vi "Add Properties.vi"(8 "error in":errorcluster, 10 "Item in":refnum<class "Item.lvclass">, 11 "Node Ptr in":T1 format="%.0x") -> (0 "error out":errorcluster, 3 "Node Ptr out":T1 format="%.0x")   [LabVIEW 2024, in "FPGA Addon System Explorer.lvlib"]
uses:
  FPGA Addon System Explorer.lvlib
  <vilib>/NI VeriStand/Custom Device API/Custom Device Item Ref.ctl
  Parser/Item/Item.lvclass
  <vilib>/NI VeriStand/Custom Device API/Dependent File Optional Info.ctl
  Parser/Property/Get Property Data/Get Property Data (Double).vi
  <vilib>/NI VeriStand/Custom Device API/Set Item Property (Double).vi
  Parser/Property/Get Property Data/Get Property Data (Boolean).vi
  <vilib>/NI VeriStand/Custom Device API/Set Item Property (Boolean).vi
  Parser/Property/Get Property Data/Get Property Data (DoubleArray).vi
  <vilib>/NI VeriStand/Custom Device API/Set Item Property (Double Array).vi
  Parser/Property/Get Property Data/Get Property Data (StringArray).vi
  <vilib>/NI VeriStand/Custom Device API/Set Item Property (String Array).vi
  Parser/Property/Get Property Data/Get Property Data (I32).vi
  <vilib>/NI VeriStand/Custom Device API/Set Item Property (I32).vi
  Parser/Property/Get Property Data/Get Property Data (U32).vi
  <vilib>/NI VeriStand/Custom Device API/Set Item Property (U32).vi
  Parser/Property/Get Property Data/Get Property Data (U16).vi
  <vilib>/NI VeriStand/Custom Device API/Set Item Property (U16).vi
  Parser/Property/Get Property Data/Get Property Data (U64).vi
  <vilib>/NI VeriStand/Custom Device API/Set Item Property (U64).vi
  Parser/Property/Get Property Data/Get Property Data (I32Array).vi
  <vilib>/NI VeriStand/Custom Device API/Set Item Property (I32 Array).vi
  Parser/Property/Get Property Data/Get Property Data (U32Array).vi
  <vilib>/NI VeriStand/Custom Device API/Set Item Property (U32 Array).vi
  Parser/Property/Get Property Data/Get Property Data (Variant).vi
  <vilib>/NI VeriStand/Custom Device API/Set Item Property (Variant).vi
  Parser/Property/Get Property Data/Get Property Data (String).vi
  <vilib>/NI VeriStand/Custom Device API/Set Item Property (String).vi
  Parser/Property/Get Property Data/Get Property Data (Path).vi
  <vilib>/NI VeriStand/Custom Device API/Set Item Property (Path).vi
  Parser/Property/Get Property Data/Get Property Data (Dictionary).vi
  Parser/Property/Get Property Data/Get Property Data (DependentFile).vi
  <vilib>/NI VeriStand/Custom Device API/Set Item Property (Dependent File).vi
  <vilib>/NI VeriStand/Custom Device API/Custom Device API.lvlib
  Parser/Property/Property.lvclass
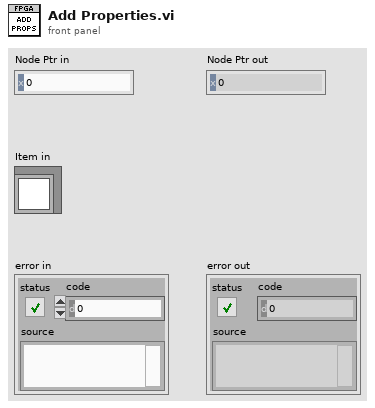
[diagram p1: front panel]
types:
  T1 = typedef "Custom Device API.lvlib/Custom Device Item Ref.ctl" = u64
  T2 = typedef "Custom Device API.lvlib/Dependent File Optional Info.ctl" = cluster{"Version":string, "RTDestination":path, "ForceDownload":bool, "SupportedTarget":string, "MD5":string}
  T3 = typedef "Parser.lvlib/Property.lvclass/Property Type.ctl" = enum16{"Boolean", "Double", "String", "Path", "Dictionary", "DependentFile", "I16", "I32", "I64", "U16", "U32", "U64", "BooleanArray", "DoubleArray", "StringArray", "I16Array", "I32Array", "I64Array", "U16Array", "U32Array", "U64Array", "Variant"}
  T4 = cluster{"Name":string, "Type":T3, "Value":variant}[]
  T5 = typedef "Parser.lvlib/Property.lvclass/DependentFile.ctl" = cluster{"Path":path, "Version":string, "RTDestination":path, "ForceDownload":bool, "SupportedTarget":string, "MD5":string, " Type":string}
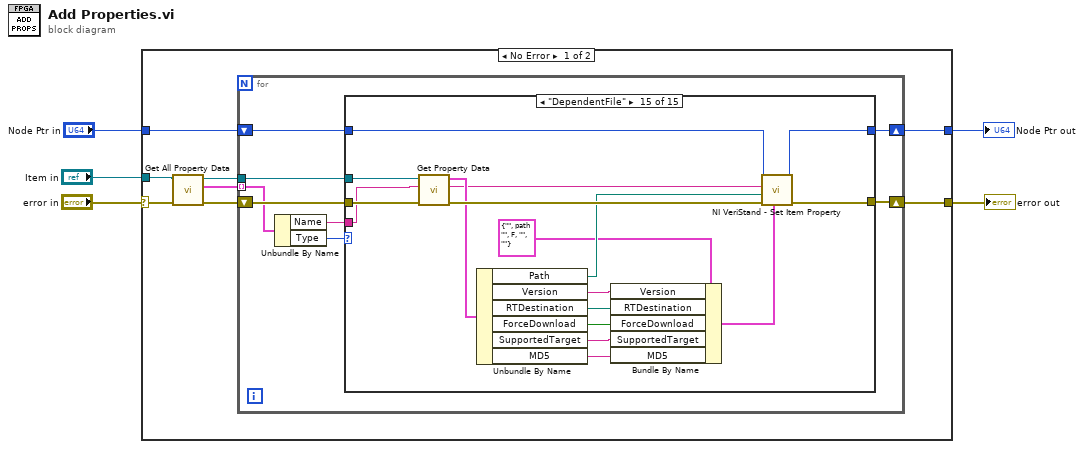
[diagram p0: block diagram]
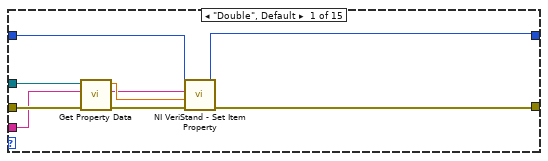
[diagram p2: hidden frame]
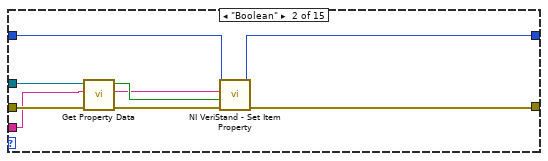
[diagram p3: hidden frame]
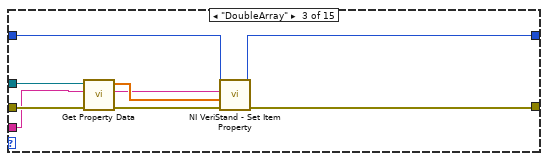
[diagram p4: hidden frame]
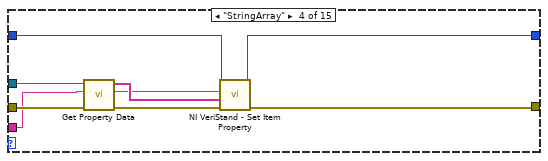
[diagram p5: hidden frame]
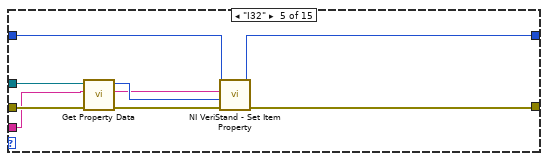
[diagram p6: hidden frame]
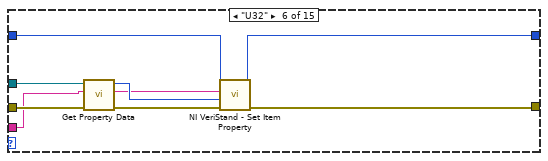
[diagram p7: hidden frame]
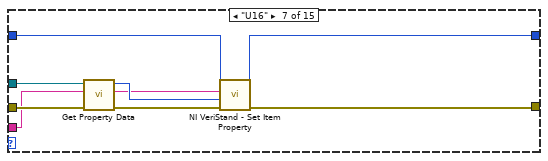
[diagram p8: hidden frame]
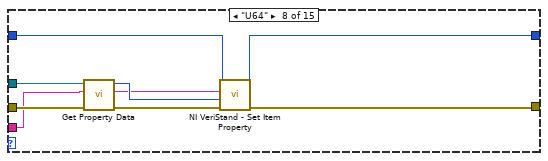
[diagram p9: hidden frame]
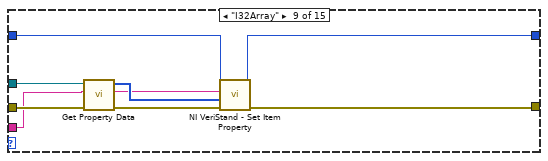
[diagram p10: hidden frame]
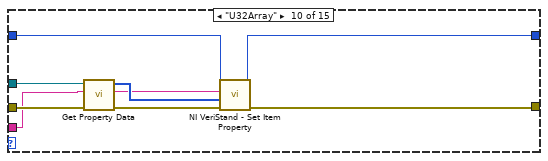
[diagram p11: hidden frame]
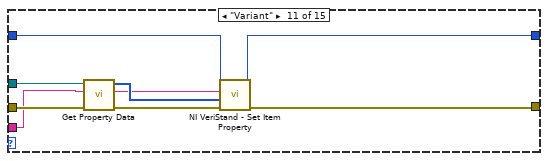
[diagram p12: hidden frame]
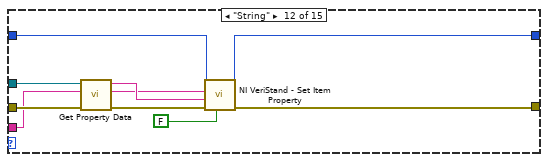
[diagram p13: hidden frame]
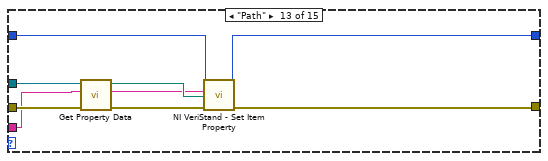
[diagram p14: hidden frame]
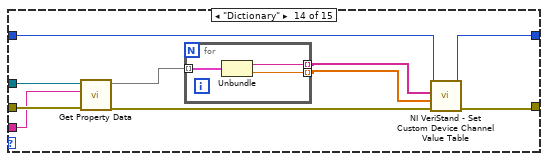
[diagram p15: hidden frame]
diagram:
  n1 = case shown="No Error" "error in" {
    selector: "error in" -> [w11 w157]
    tunnel: "Node Ptr in" -> [w10 w156]
    tunnel: "Item in" -> [w6 _]
    tunnel: [w12 w157] -> w4
    tunnel: [w9 w156] -> w1
    frame No Error {
      n2 = call "Get All Property Data.vi"("error in"=w11, "Item in"=w6) -> ("error out"=w13:errorcluster, "Properties Data"=w8:T4, "Item out"=w7:refnum<class "Item.lvclass">)  [unwired: 7 in]
      n3 = for {
        tunnel: w7 -> [w19]
        shift-right: [w20] -> w12
        shift-left: w13 -> [w21]
        shift-right: [w17] -> w9
        shift-left: w10 -> [w18]
        tunnel: w8 -> [w16] mode=indexing
        n4 = Unbundle By Name(w16) -> ("Name"=w14:string, "Type"=w15:T3)
        n5 = case shown="\"DependentFile\"" w15 {
          tunnel: w19 -> [w26 w34 w42 w50 w58 w66 w74 w82 w90 w98 w106 w115 w123 w133 w142]
          tunnel: w21 -> [w29 w37 w45 w53 w61 w69 w77 w85 w93 w101 w109 w118 w126 w136 w155]
          tunnel: [w27 w35 w43 w51 w59 w67 w75 w83 w91 w99 w107 w116 w124 w135 w153] -> w20
          tunnel: w18 -> [w25 w33 w41 w49 w57 w65 w73 w81 w89 w97 w105 w114 w122 w132 w152]
          tunnel: [w23 w31 w39 w47 w55 w63 w71 w79 w87 w95 w103 w111 w120 w128 w141] -> w17
          tunnel: w14 -> [w22 w30 w38 w46 w54 w62 w70 w78 w86 w94 w102 w110 w119 w127 w140]
          frame "Double", Default {
            n6 = call-poly "Get Property Data.vi"("error in"=w29, "Property Name"=w22, "Item in"=w26) -> ("error out"=w28:errorcluster, "Property Value"=w24:dbl)  [unwired: 7 in]
            n7 = call-poly <vilib>:"NI VeriStand - Set Item Property.vi"("error in (no error)"=w28, "Value"=w24, "Property Name"=w22, "Item Ref in"=w25) -> ("error out"=w27:errorcluster, "Item Ref out"=w23:T1)  [unwired: 5 in, 1 out]
          }
          frame "Boolean" {
            n8 = call-poly "Get Property Data.vi"("error in"=w37, "Property Name"=w30, "Item in"=w34) -> ("error out"=w36:errorcluster, "Property Value"=w32:bool)  [unwired: 7 in]
            n9 = call-poly <vilib>:"NI VeriStand - Set Item Property.vi"("error in (no error)"=w36, "Value"=w32, "Property Name"=w30, "Item Ref in"=w33) -> ("error out"=w35:errorcluster, "Item Ref out"=w31:T1)  [unwired: 5 in, 1 out]
          }
          frame "DoubleArray" {
            n10 = call-poly "Get Property Data.vi"("error in"=w45, "Property Name"=w38, "Item in"=w42) -> ("error out"=w44:errorcluster, "Property Value"=w40:dbl[])  [unwired: 7 in]
            n11 = call-poly <vilib>:"NI VeriStand - Set Item Property.vi"("error in (no error)"=w44, "Value"=w40, "Property Name"=w38, "Item Ref in"=w41) -> ("error out"=w43:errorcluster, "Item Ref out"=w39:T1)  [unwired: 5 in, 1 out]
          }
          frame "StringArray" {
            n12 = call-poly "Get Property Data.vi"("error in"=w53, "Property Name"=w46, "Item in"=w50) -> ("error out"=w52:errorcluster, "Property Value"=w48:string[])  [unwired: 7 in]
            n13 = call-poly <vilib>:"NI VeriStand - Set Item Property.vi"("error in (no error)"=w52, "Value"=w48, "Property Name"=w46, "Item Ref in"=w49) -> ("error out"=w51:errorcluster, "Item Ref out"=w47:T1)  [unwired: 5 in, 1 out]
          }
          frame "I32" {
            n14 = call-poly "Get Property Data.vi"("error in"=w61, "Property Name"=w54, "Item in"=w58) -> ("error out"=w60:errorcluster, "Property Value"=w56:i32)  [unwired: 7 in]
            n15 = call-poly <vilib>:"NI VeriStand - Set Item Property.vi"("error in (no error)"=w60, "Value"=w56, "Property Name"=w54, "Item Ref in"=w57) -> ("error out"=w59:errorcluster, "Item Ref out"=w55:T1)  [unwired: 5 in, 1 out]
          }
          frame "U32" {
            n16 = call-poly "Get Property Data.vi"("error in"=w69, "Property Name"=w62, "Item in"=w66) -> ("error out"=w68:errorcluster, "Property Value"=w64:u32)  [unwired: 7 in]
            n17 = call-poly <vilib>:"NI VeriStand - Set Item Property.vi"("error in (no error)"=w68, "Value"=w64, "Property Name"=w62, "Item Ref in"=w65) -> ("error out"=w67:errorcluster, "Item Ref out"=w63:T1)  [unwired: 5 in, 1 out]
          }
          frame "U16" {
            n18 = call-poly "Get Property Data.vi"("error in"=w77, "Property Name"=w70, "Item in"=w74) -> ("error out"=w76:errorcluster, "Property Value"=w72:u16)  [unwired: 7 in]
            n19 = call-poly <vilib>:"NI VeriStand - Set Item Property.vi"("error in (no error)"=w76, "Value"=w72, "Property Name"=w70, "Item Ref in"=w73) -> ("error out"=w75:errorcluster, "Item Ref out"=w71:T1)  [unwired: 5 in, 1 out]
          }
          frame "U64" {
            n20 = call-poly "Get Property Data.vi"("error in"=w85, "Property Name"=w78, "Item in"=w82) -> ("error out"=w84:errorcluster, "Property Value"=w80:u64)  [unwired: 7 in]
            n21 = call-poly <vilib>:"NI VeriStand - Set Item Property.vi"("error in (no error)"=w84, "Value"=w80, "Property Name"=w78, "Item Ref in"=w81) -> ("error out"=w83:errorcluster, "Item Ref out"=w79:T1)  [unwired: 5 in, 1 out]
          }
          frame "I32Array" {
            n22 = call-poly "Get Property Data.vi"("error in"=w93, "Property Name"=w86, "Item in"=w90) -> ("error out"=w92:errorcluster, "Property Value"=w88:i32[])  [unwired: 7 in]
            n23 = call-poly <vilib>:"NI VeriStand - Set Item Property.vi"("error in (no error)"=w92, "Value"=w88, "Property Name"=w86, "Item Ref in"=w89) -> ("error out"=w91:errorcluster, "Item Ref out"=w87:T1)  [unwired: 5 in, 1 out]
          }
          frame "U32Array" {
            n24 = call-poly "Get Property Data.vi"("error in"=w101, "Property Name"=w94, "Item in"=w98) -> ("error out"=w100:errorcluster, "Property Value"=w96:u32[])  [unwired: 7 in]
            n25 = call-poly <vilib>:"NI VeriStand - Set Item Property.vi"("error in (no error)"=w100, "Value"=w96, "Property Name"=w94, "Item Ref in"=w97) -> ("error out"=w99:errorcluster, "Item Ref out"=w95:T1)  [unwired: 5 in, 1 out]
          }
          frame "Variant" {
            n26 = call-poly "Get Property Data.vi"("error in"=w109, "Property Name"=w102, "Item in"=w106) -> ("error out"=w108:errorcluster, "Property Value"=w104:u8[])  [unwired: 7 in]
            n27 = call-poly <vilib>:"NI VeriStand - Set Item Property.vi"("error in (no error)"=w108, "Value"=w104, "Property Name"=w102, "Item Ref in"=w105) -> ("error out"=w107:errorcluster, "Item Ref out"=w103:T1)  [unwired: 5 in, 1 out]
          }
          frame "String" {
            n28 = call-poly "Get Property Data.vi"("error in"=w118, "Property Name"=w110, "Item in"=w115) -> ("error out"=w117:errorcluster, "Property Value"=w113:string)  [unwired: 7 in]
            n29 = call-poly <vilib>:"NI VeriStand - Set Item Property.vi"("Binary String (T)"=FALSE, "error in (no error)"=w117, "Value"=w113, "Property Name"=w110, "Item Ref in"=w114) -> ("error out"=w116:errorcluster, "Item Ref out"=w111:T1)  [unwired: 4 in, 1 out]
          }
          frame "Path" {
            n30 = call-poly "Get Property Data.vi"("error in"=w126, "Property Name"=w119, "Item in"=w123) -> ("error out"=w125:errorcluster, "Property Value"=w121:path)  [unwired: 7 in]
            n31 = call-poly <vilib>:"NI VeriStand - Set Item Property.vi"("error in (no error)"=w125, "Value"=w121, "Property Name"=w119, "Item Ref in"=w122) -> ("error out"=w124:errorcluster, "Item Ref out"=w120:T1)  [unwired: 5 in, 1 out]
          }
          frame "Dictionary" {
            n32 = call-poly "Get Property Data.vi"("error in"=w136, "Property Name"=w127, "Item in"=w133) -> ("error out"=w134:errorcluster, "Property Value"=w131:map{string, dbl})  [unwired: 7 in]
            n33 = for {
              tunnel: w131 -> [w139] mode=indexing
              tunnel: [w138] -> w130 mode=indexing
              tunnel: [w137] -> w129 mode=indexing
              n34 = Unbundle(w139) -> (w138:string, w137:dbl)
            }
            n35 = call <vilib>:"NI VeriStand - Set Custom Device Channel Value Table.vi"("error in (no error)"=w134, "Values"=w129, "Names"=w130, "Channel Ref in"=w132) -> ("error out"=w135:errorcluster, "Channel Ref out"=w128:T1)  [unwired: 6 in]
          }
          frame "DependentFile" {
            n36 = call-poly "Get Property Data.vi"("error in"=w155, "Property Name"=w140, "Item in"=w142) -> ("error out"=w154:errorcluster, "Property Value"=w151:T5)  [unwired: 7 in]
            n37 = Unbundle By Name(w151) -> ("Path"=w150:path, "Version"=w148:string, "RTDestination"=w147:path, "ForceDownload"=w146:bool, "SupportedTarget"=w145:string, "MD5"=w144:string)
            n38 = Bundle By Name(cluster=T2 {"Version"="", "RTDestination"=path "", "ForceDownload"=FALSE, "SupportedTarget"="", "MD5"=""} ("OptionalInfo"), "Version"=w148, "RTDestination"=w147, "ForceDownload"=w146, "SupportedTarget"=w145, "MD5"=w144) -> (w143:T2)
            n39 = call-poly <vilib>:"NI VeriStand - Set Item Property.vi"("OptionalInfo"=w143, "error in (no error)"=w154, "Path"=w150, "Property Name"=w140, "Item Ref in"=w152) -> ("error out"=w153:errorcluster, "Item Ref out"=w141:T1)  [unwired: 4 in, 1 out]
          }
        }
      }
    }
    frame Error {
    }
  }
  "error out" <- w4
  "Node Ptr out" <- w1
